vi "Error_Handler_EHL_FGV.vi"(8 "error in (no error)":errorcluster, 10 "Ignore Errors (Runtime)":i32[](array[numeric]), 11 "queue in":refnum<queue>) -> (0 "error Out":errorcluster)   [LabVIEW 2024, in "Multicom_MP711134-14V.lvlib"]
doc: "This VI\n---------------------------------------------------------\nMessage_Loop_Handler_FGV.\n---------------------------------------------------------\n-Handels the error occured in message handling loop"
uses:
  Multicom_MP711134-14V.lvlib
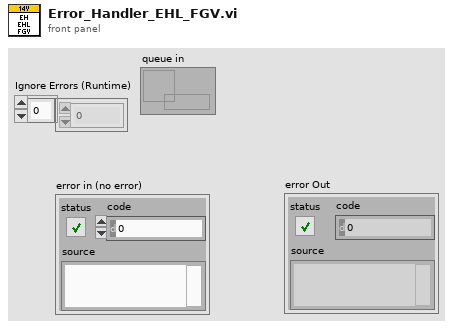
[diagram p1: front panel]
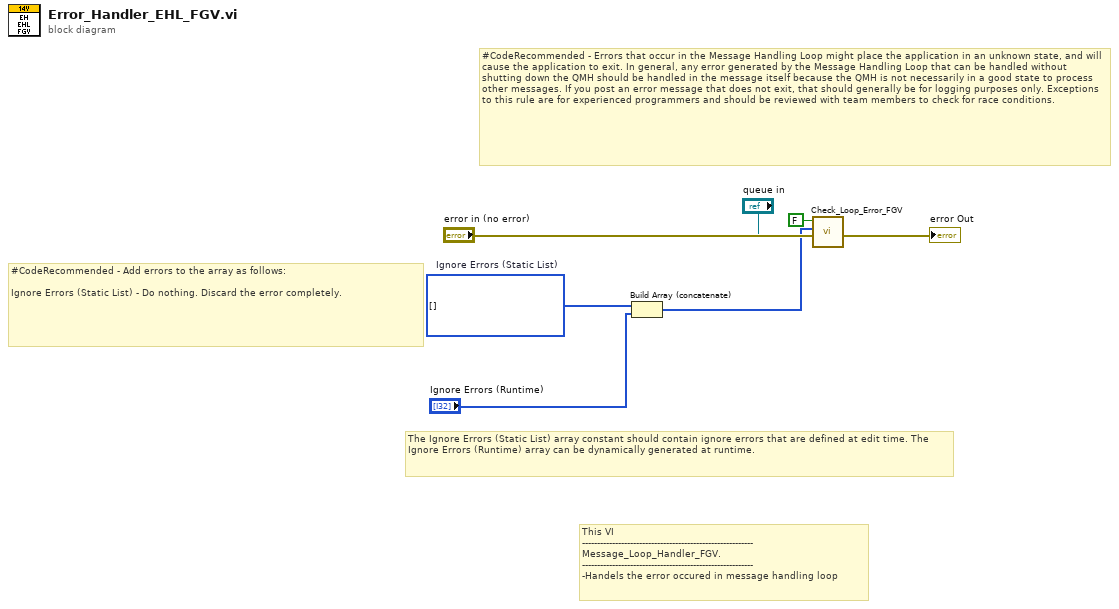
[diagram p0: block diagram]
diagram:
  w2 = i32[] []  # Ignore Errors (Static List)
  # "This VI\n---------------------------------------------------------\nMessage_Loop_Handler_FGV.\n---------------------------------------------------------\n-Handels the error occured in message handling loop"
  # "#CodeRecommended - Errors that occur in the Message Handling Loop might place the application in an unknown state, and will cause the application to exit. In general, any error generated by the Message Handling Loop that can be handled without shutting down the QMH should be handled in the message itself because the QMH is not necessarily in a good state to process other messages. If you post an error message that does not exit, that should generally be for logging purposes only. Exceptions to this rule are for experienced programmers and should be reviewed with team members to check for race conditions."
  # "The Ignore Errors (Static List) array constant should contain ignore errors that are defined at edit time. The Ignore Errors (Runtime) array can be dynamically generated at runtime."
  # "#CodeRecommended - Add errors to the array as follows:\n\nIgnore Errors (Static List) - Do nothing. Discard the error completely."
  n1 = Build Array (concatenate)(w2, "Ignore Errors (Runtime)") -> (w5:i32[])
  n2 = call "Check_Loop_Error_FGV.vi"("error in (no error)"="error in (no error)", "queue in"="queue in", "Ignore Errors"=w5, "Exit on Error? (F)"=FALSE) -> ()  [unwired: 7 in, 1 out]
  "error Out" <- "error in (no error)"
